vi "Washing_Machine.vi"() -> ()   [LabVIEW 2023]
doc: "This is the main vi that simulates the washing machine."
uses:
  Controls/Wash_Type.ctl
  Controls/Sequence_Display.ctl
  Controls/Washing_Data.ctl
  Controls/Queue_Operation_Select.ctl
  Controls/State_and_Data.ctl
  Controls/Timer_Operation_Select.ctl
  Controls/INI_Operation_Select.ctl
panel:
  out "Sequence":T1
  out "Elapsed_Time":dbl caption="Elapsed Time"
  out "Machine_Underweight":bool
  out "Machine_Overweight":bool
  out "Machine_Load":dbl(slide) caption="Machine Load" scale=0.0..15.0
  in  "Unload":bool
  in  "Stop_Wash":bool caption="Stop Wash"
  in  "Start_Wash":bool caption="Start Wash"
  in  "Wash_Type":T2 caption="Wash Type" scale=0.0..2.0
  in  "Add_Clothes":bool
  in  "Clothes [Kg]":dbl min=0.0 max=15.0
  out "Error_Out":errorcluster
  in  "Error_In":errorcluster
  # "Load Status"
  # "Sec"
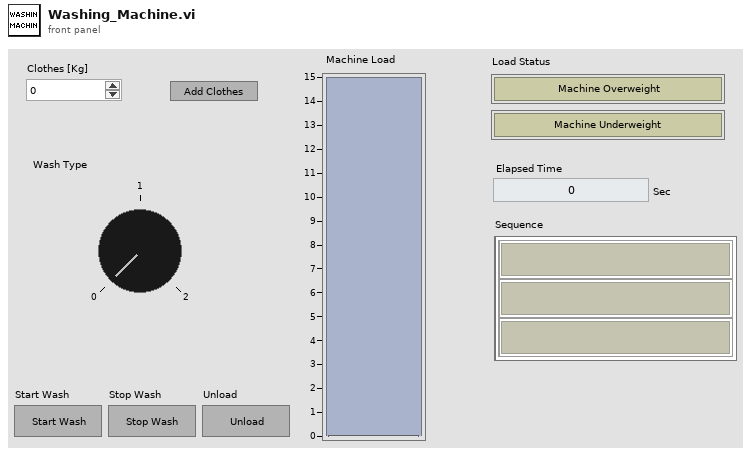
[diagram p1: front panel]
types:
  T1 = typedef "Sequence_Display.ctl" = cluster{"Sequence_LED":bool[], "Sequence_Label":string[]}
  T2 = typedef "Wash_Type.ctl" = i32
  T3 = typedef "Queue_Operation_Select.ctl" = enum16{"Obtain_Queue", "Enqueue", "Enqueue_First", "Enqueue_N", "Lossy_Enqueue", "Preview", "Queue_Status", "Dequeue", "Flush", "Release_Queue"}
  T4 = typedef "State_and_Data.ctl" = cluster{"State":string, "Data":variant}
  T5 = typedef "Washing_Data.ctl" = cluster{"Machine_Load":dbl, "Machine_Overweight":bool, "Machine_Underweight":bool, "Sequence":bool[], "Washing_Complete?":bool, "Disabled":enum8{"Enabled", "Disabled", "Disabled and Grayed Out"}, "Wash_Type":string, "Washing_Process":string[], "Process_Time":dbl[], "CSV_File_Path":path, "Current_Washing_Stage":i32, "Start?":bool, "Total_Washing_Stage":i32, "Washing_Process_F":bool[], "Machine_Load_Added":bool, "Wash_Completed_Time":dbl, "Sequence 2":T1}
  T6 = enum8{"Enabled", "Disabled", "Disabled and Grayed Out"}
  T7 = typedef "INI_Operation_Select.ctl" = enum16{"Initialize", "Read", "Read_Key", "Write"}
  T8 = typedef "Timer_Operation_Select.ctl" = enum16{"Start_Timer", "Time_Out?", "Pause_Timer", "Stop_Timer"}
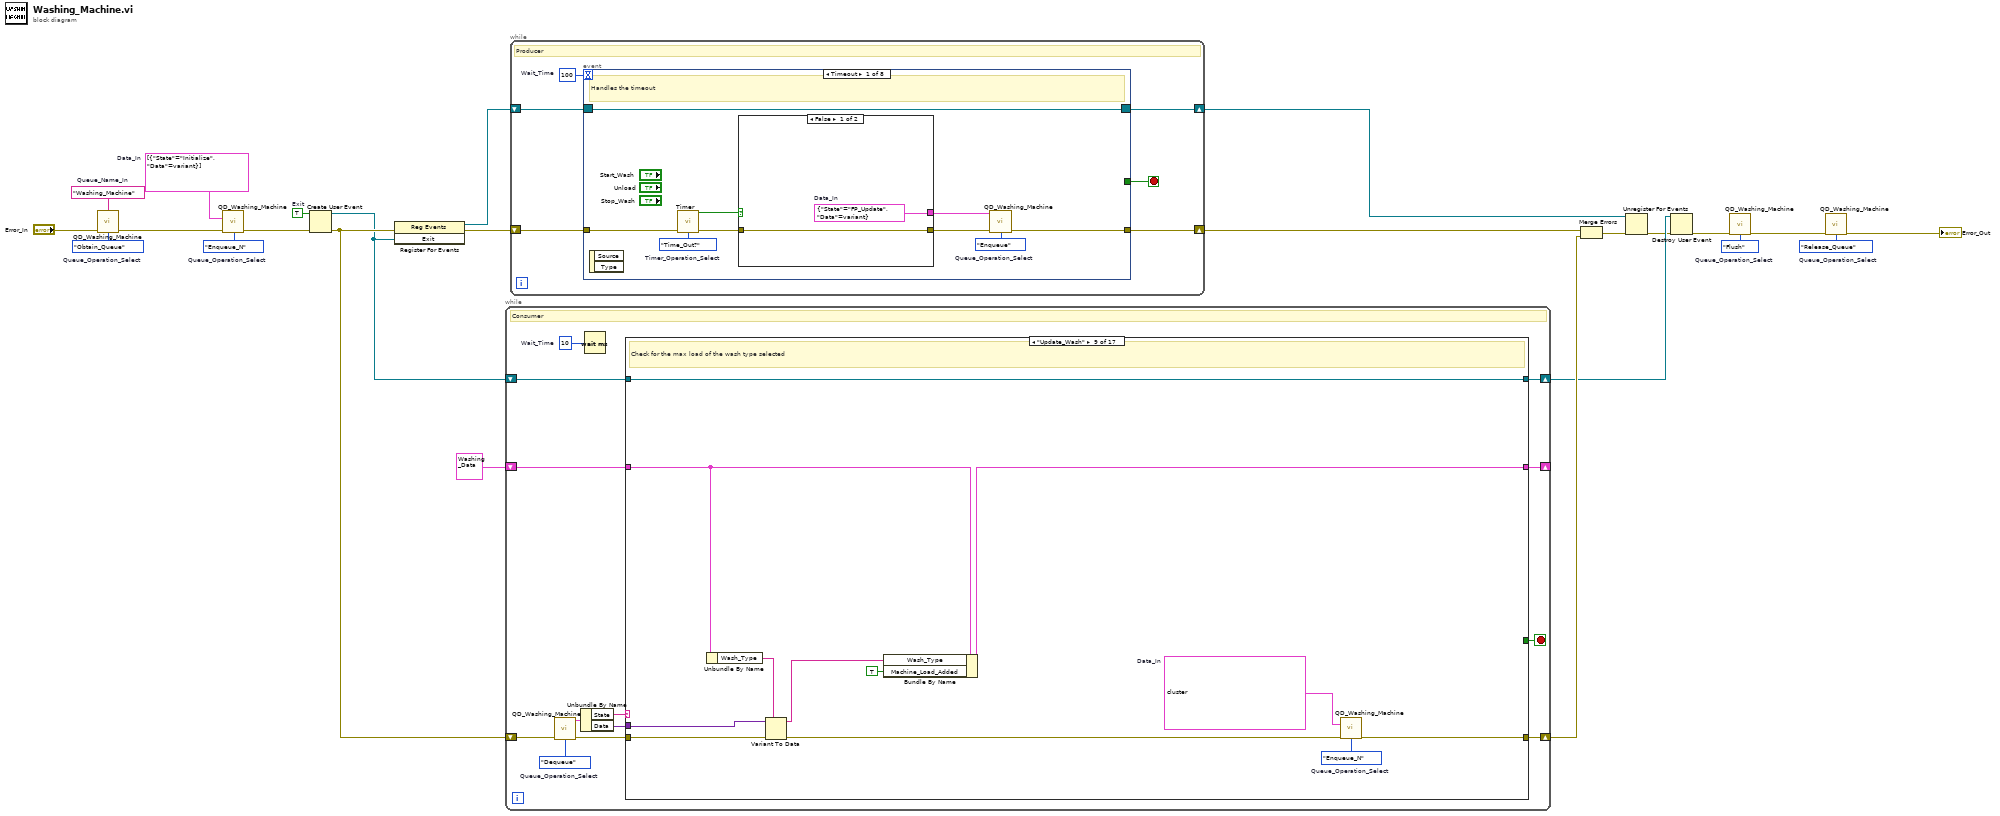
[diagram p0: block diagram]
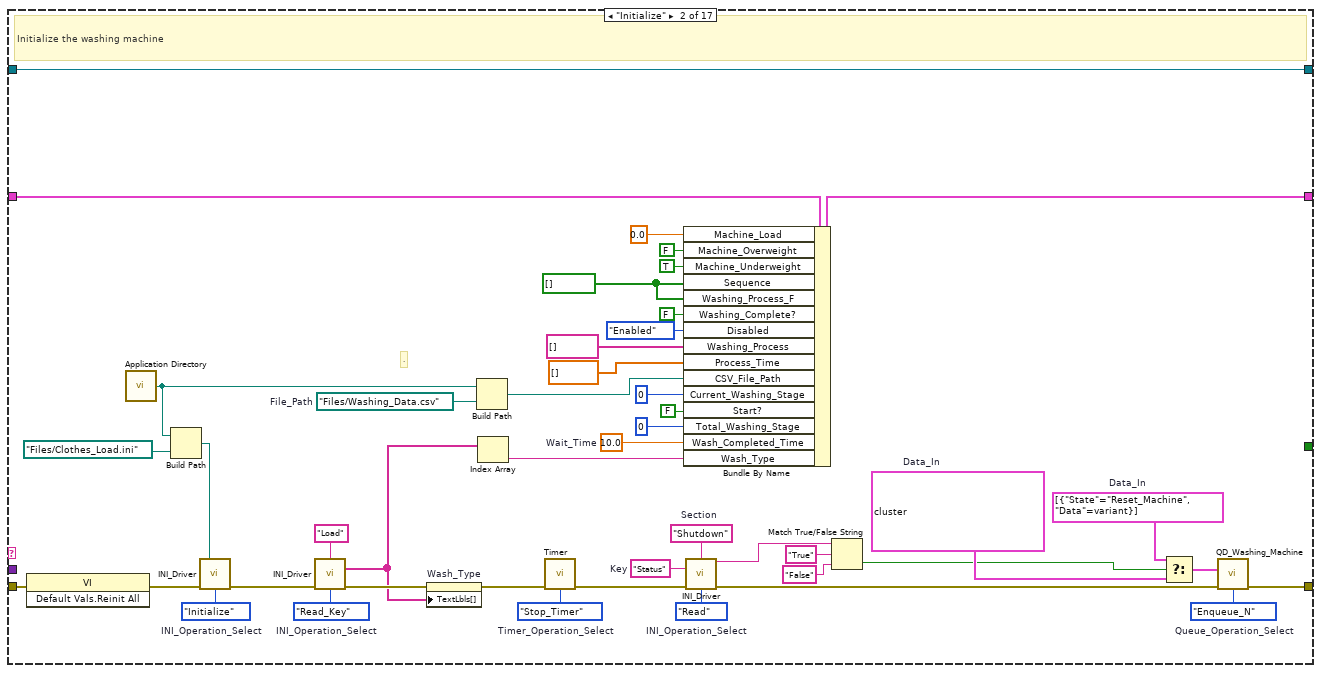
[diagram p3: hidden frame]
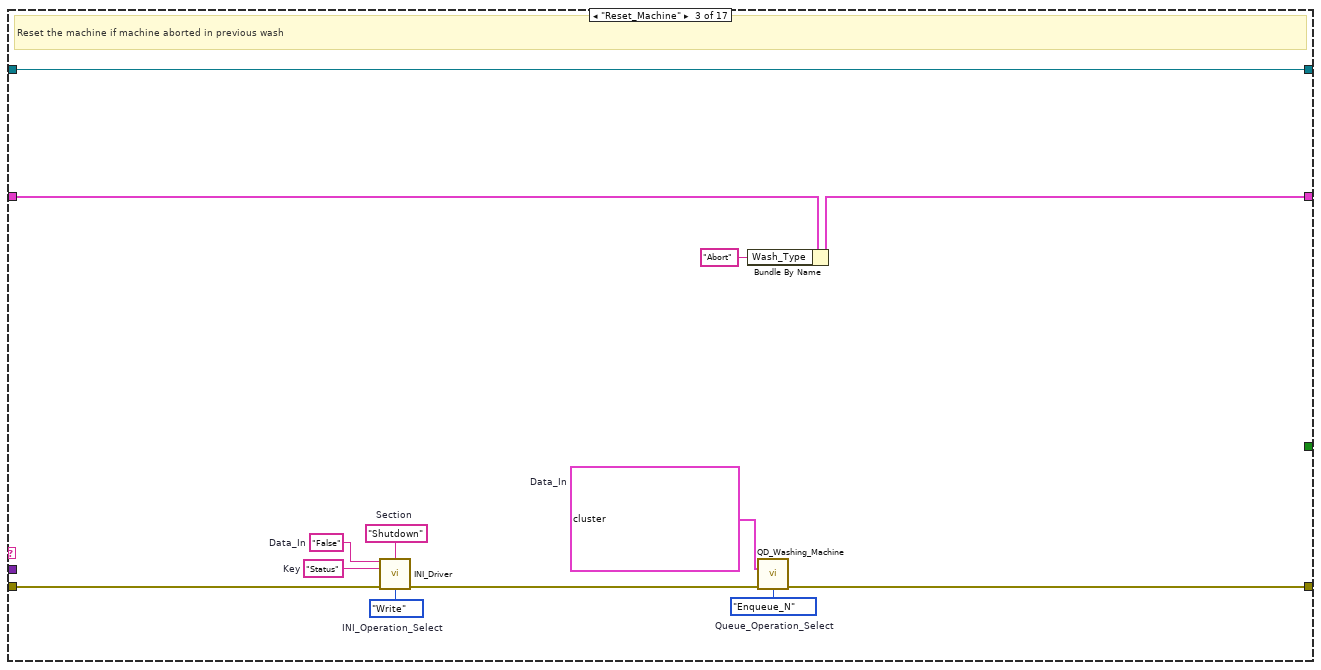
[diagram p4: hidden frame]
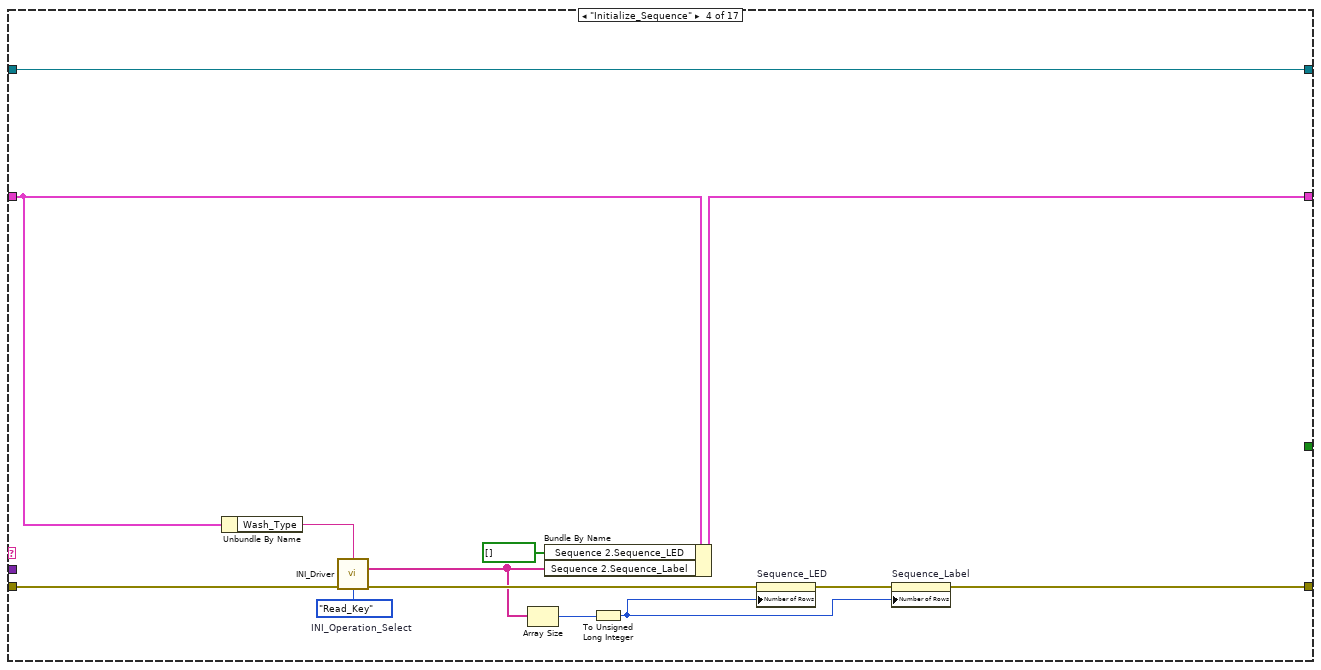
[diagram p5: hidden frame]
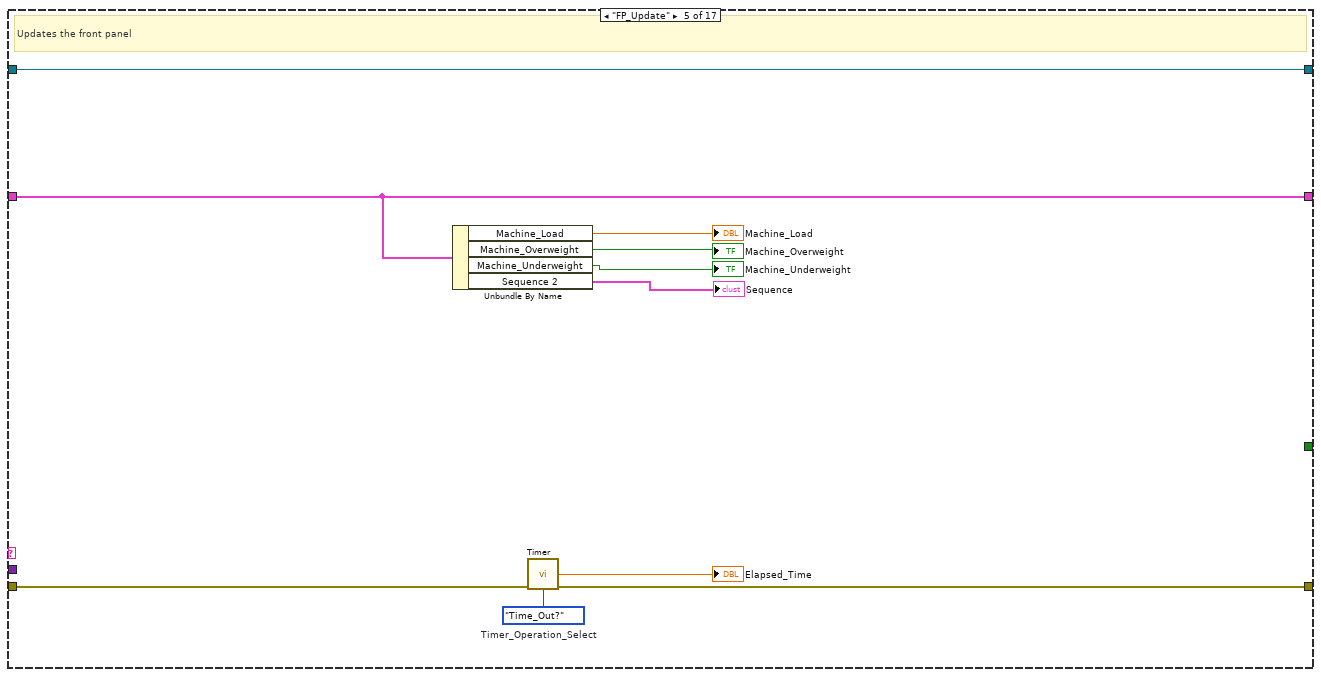
[diagram p6: hidden frame]
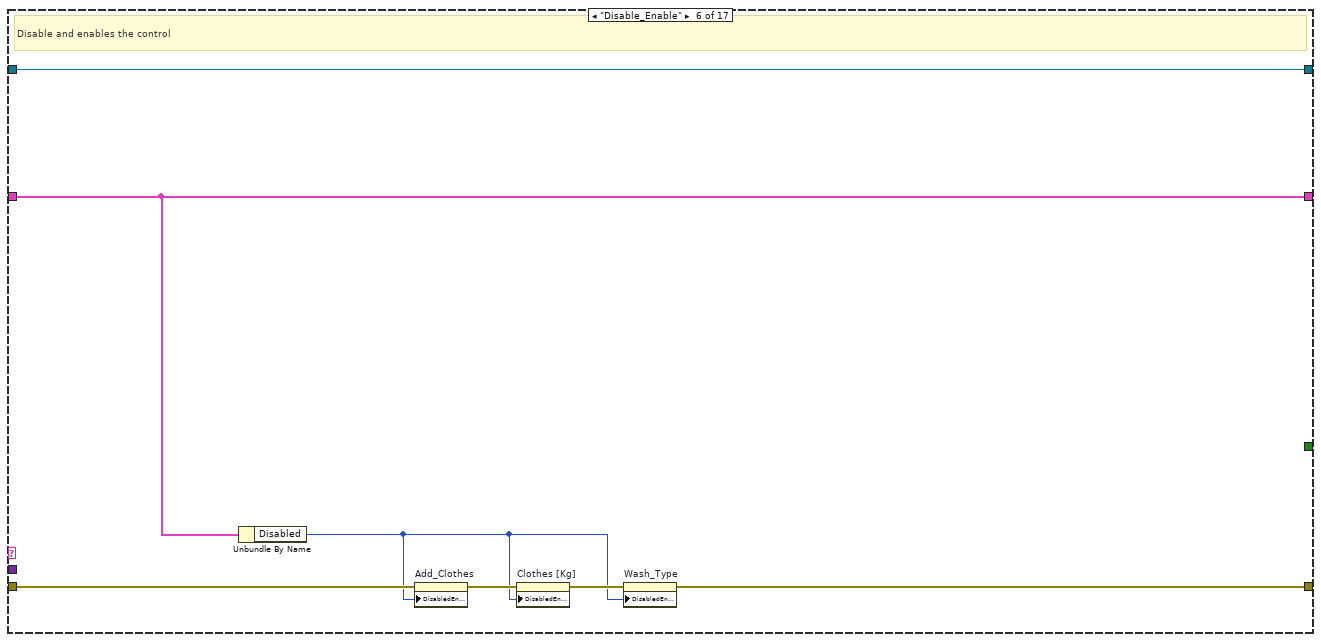
[diagram p7: hidden frame]
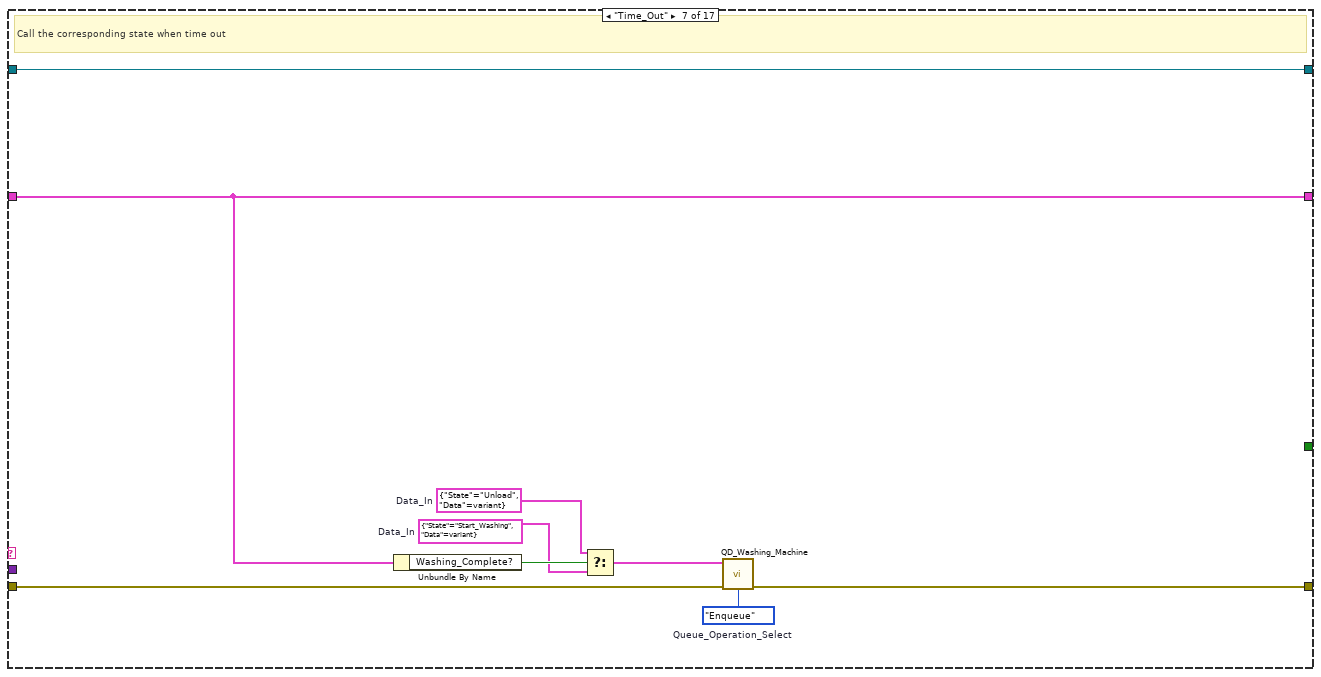
[diagram p8: hidden frame]
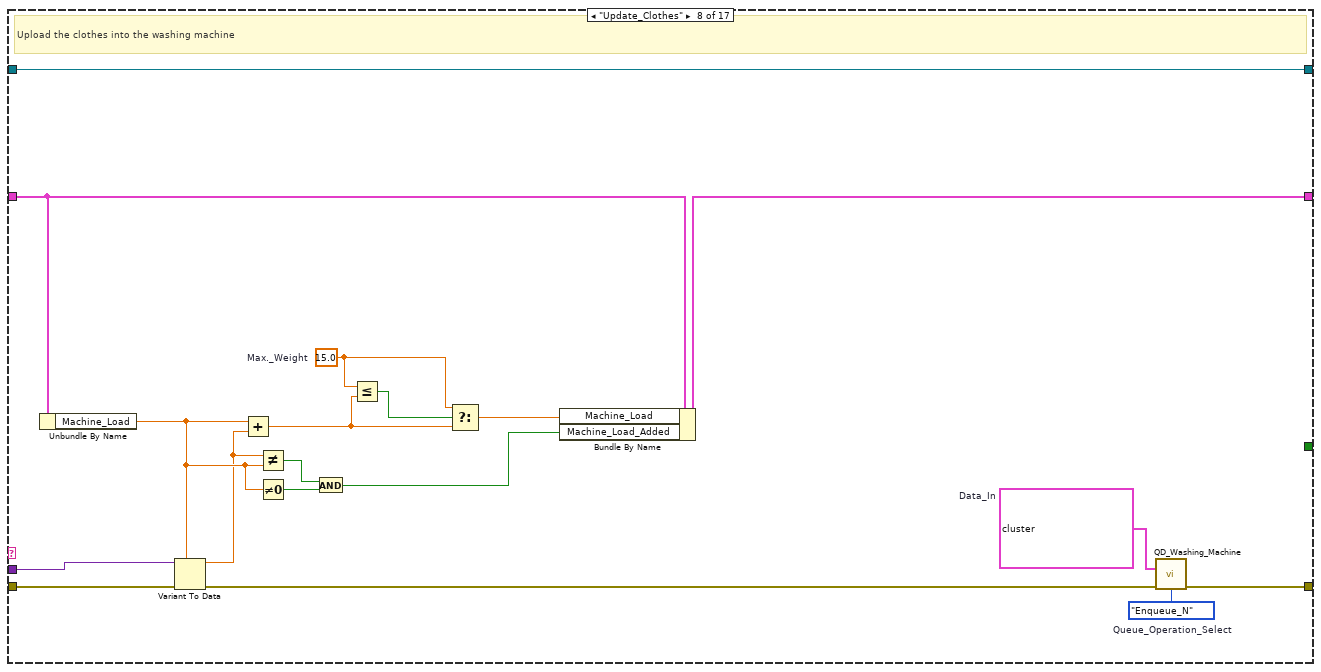
[diagram p9: hidden frame]
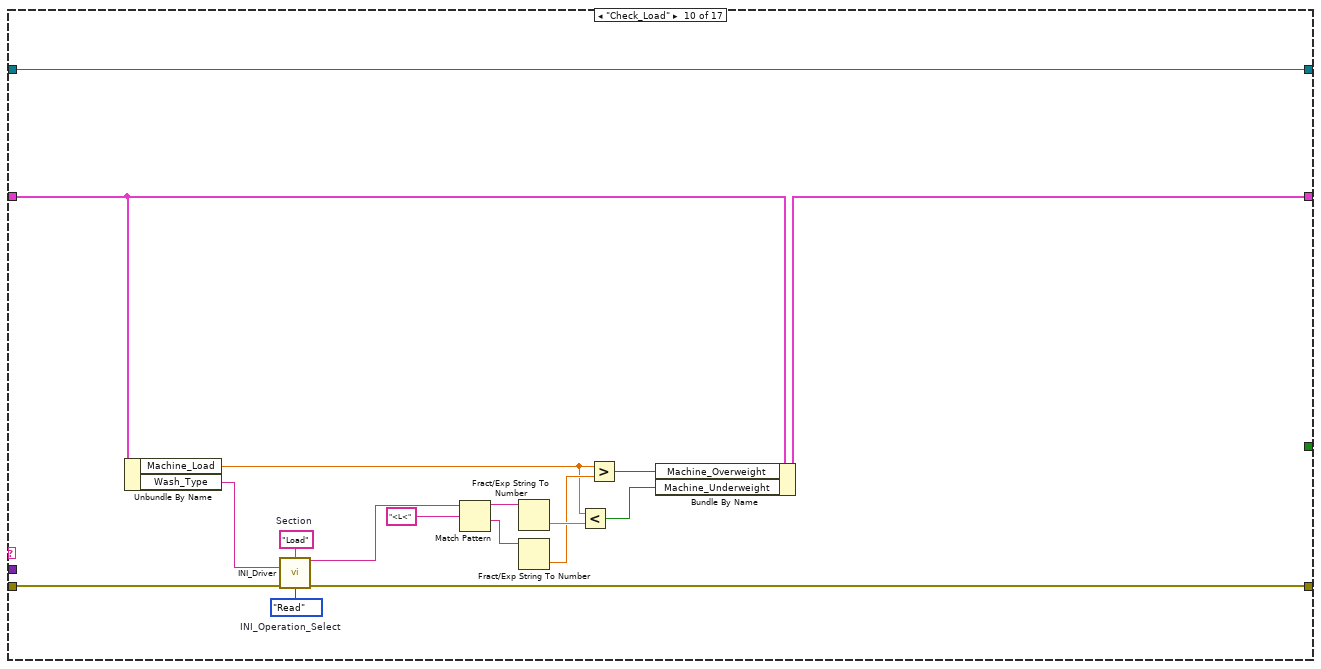
[diagram p10: hidden frame]
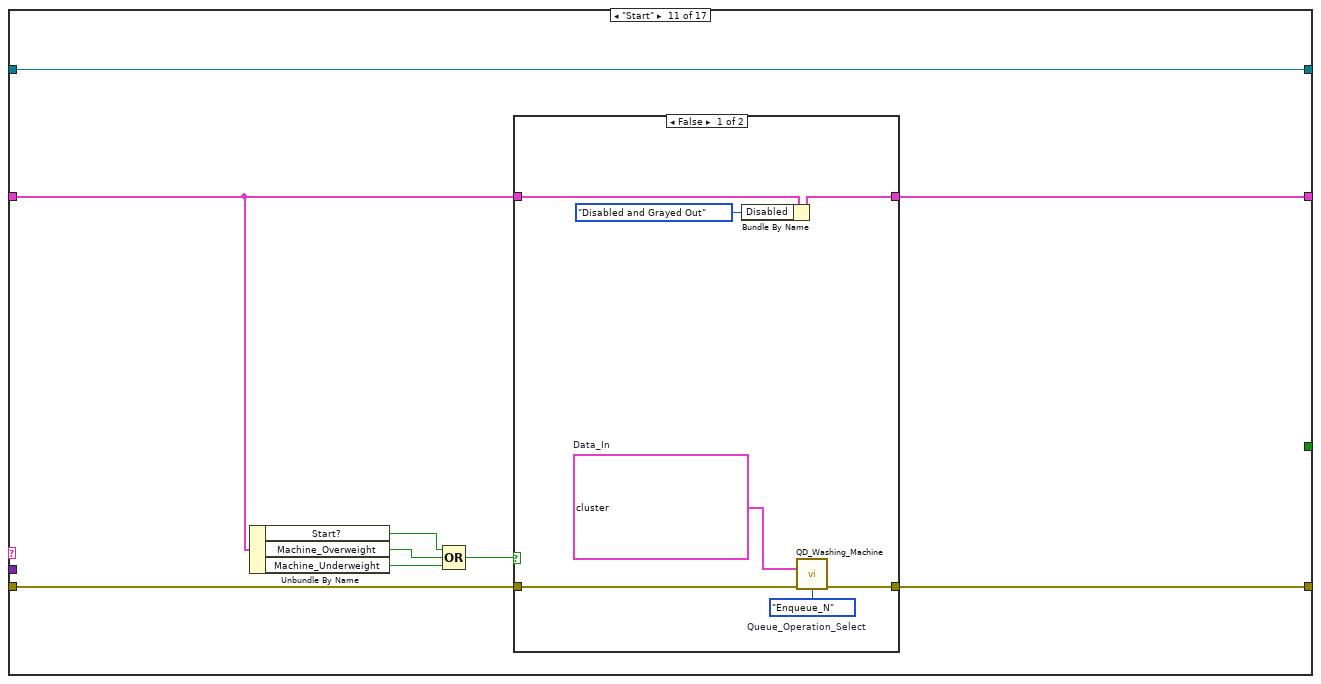
[diagram p11: hidden frame]
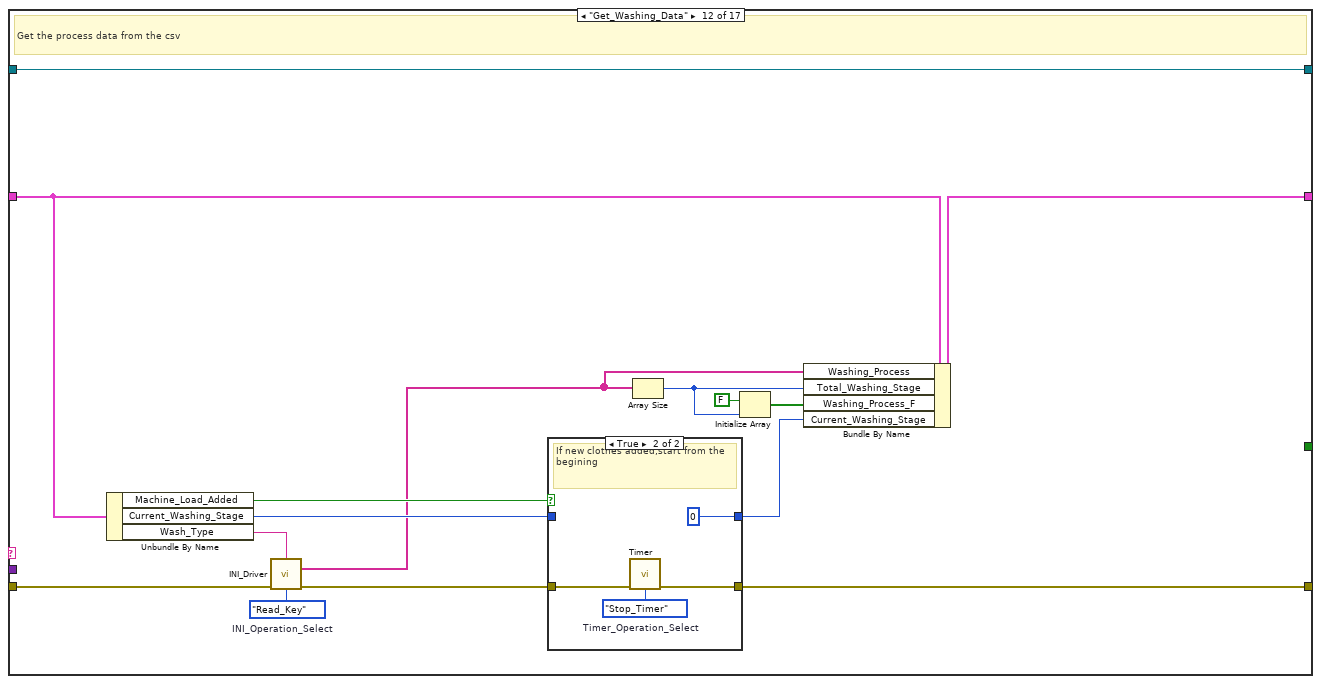
[diagram p13: hidden frame]
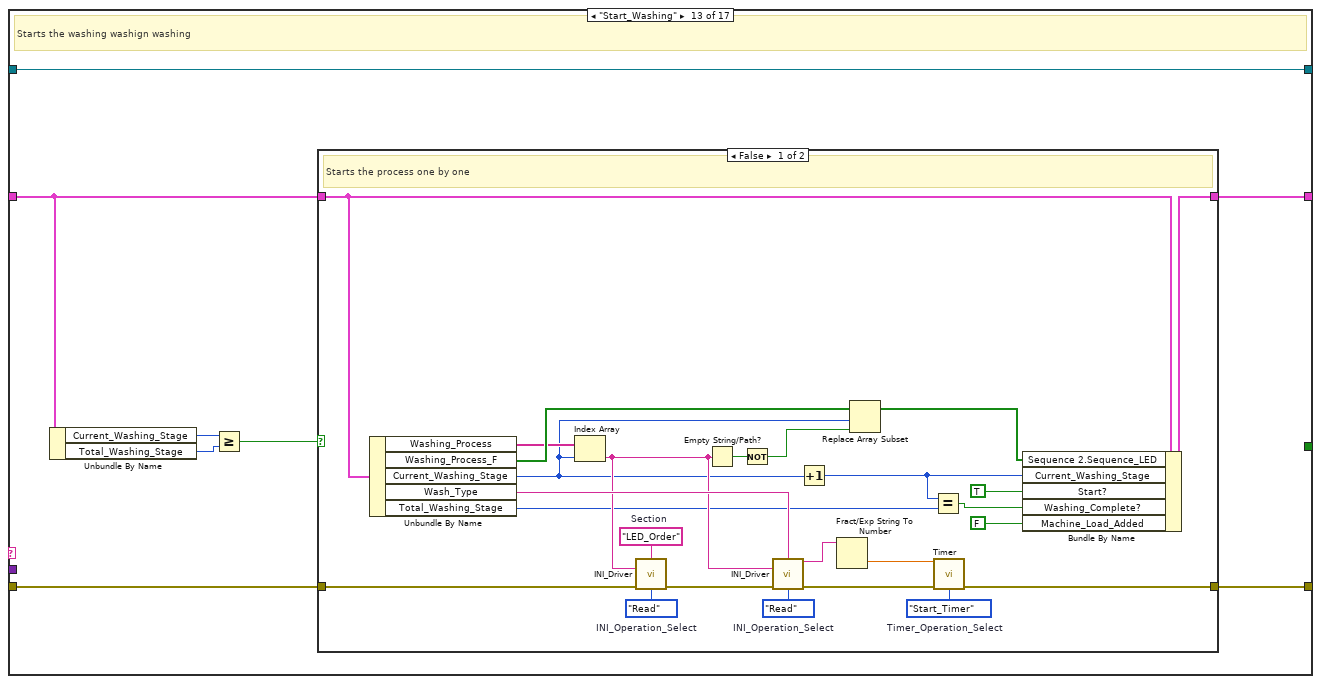
[diagram p15: hidden frame]
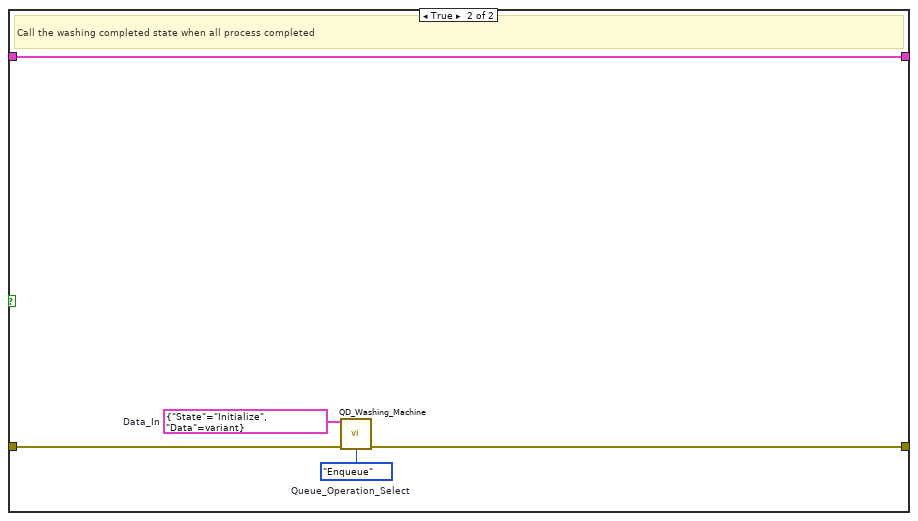
[diagram p16: hidden frame]
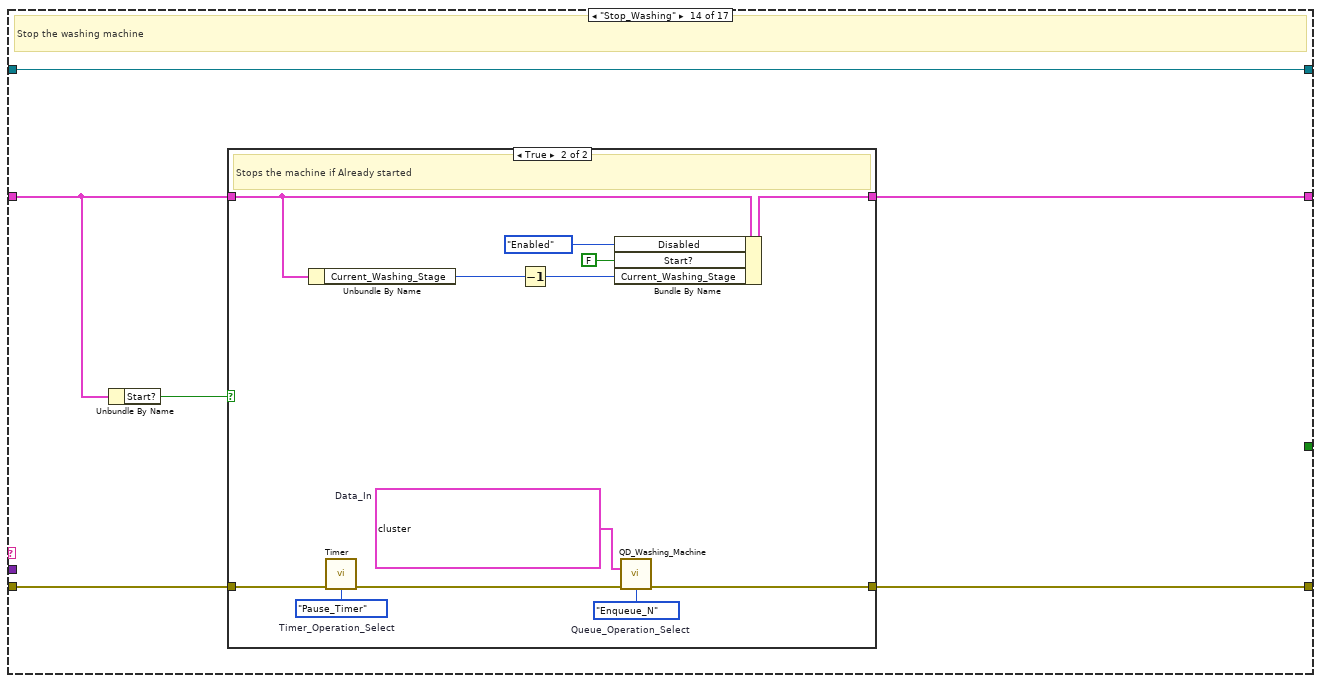
[diagram p17: hidden frame]
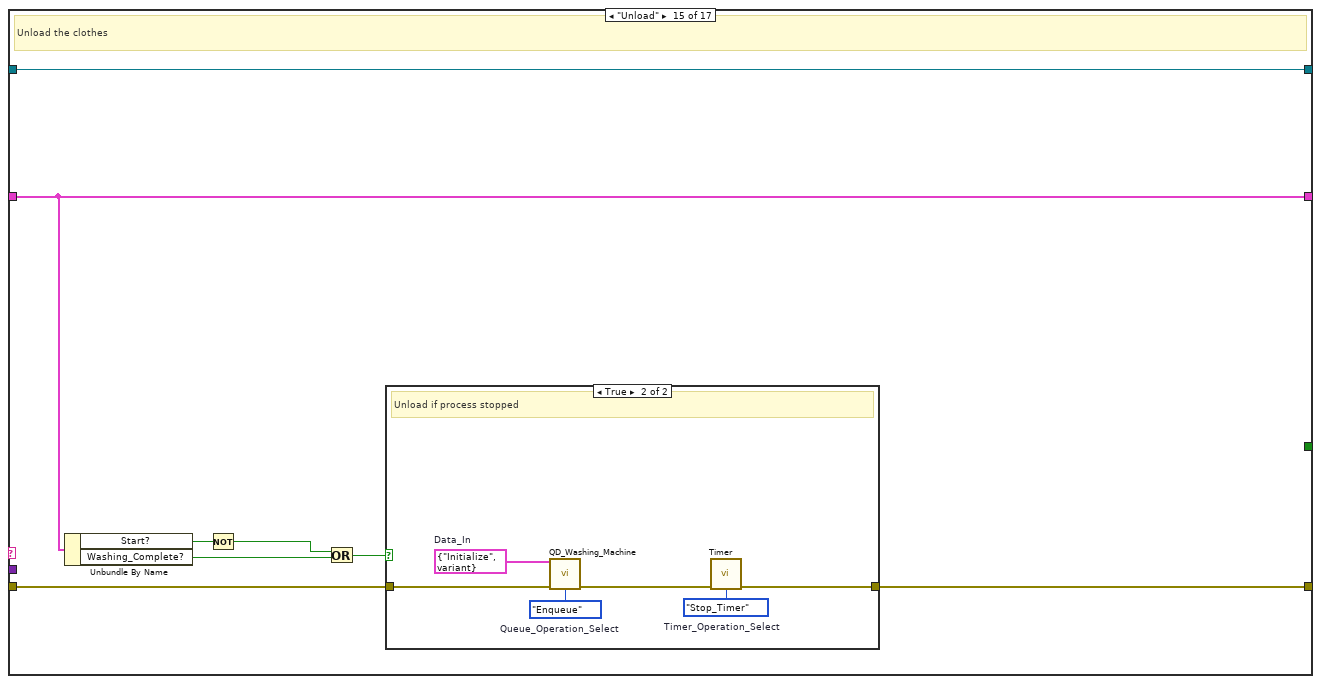
[diagram p19: hidden frame]
diagram:
  w5 = Queue_Operation_Select."Release_Queue"  # Queue_Operation_Select
  w6 = Queue_Operation_Select."Flush"  # Queue_Operation_Select
  w13 = TRUE  # Exit
  w17 = T4[] [{"State"="Initialize", "Data"=variant}]  # Data_In
  w18 = Queue_Operation_Select."Enqueue_N"  # Queue_Operation_Select
  w19 = "Washing_Machine"  # Queue_Name_In
  w20 = Queue_Operation_Select."Obtain_Queue"  # Queue_Operation_Select
  n1 = call "QD_Washing_Machine.vi"("Queue_Name_In"=w19, "Error_In"="Error_In", "Queue_Operation_Select"=w20) -> ("Error_Out"=w22:errorcluster)  [unwired: 10 in, 2 out]
  n2 = call "QD_Washing_Machine.vi"("Data_In"=w17, "Error_In"=w22, "Queue_Operation_Select"=w18) -> ("Error_Out"=w15:errorcluster)  [unwired: 10 in, 2 out]
  n3 = Create User Event(user event datatype=w13, error in=w15) -> (user event=w4:refnum<user-event>, error out=w14:errorcluster)
  n4 = register-events(error in=w14, w4) -> (reference out=w11:refnum<event-registration>, error out=w12:errorcluster)  [unwired: 1 in]
  n5 = while {
    shift-right: [w36] -> w16
    shift-left: w14 -> [w37]
    shift-right: [w30] -> _
    shift-left: T5 {"Machine_Load"=0.0, "Machine_Overweight"=FALSE, "Machine_Underweight"=FALSE, "Sequence"=[], "Washing_Complete?"=FALSE, "Disabled"=enum."Enabled", "Wash_Type"="", "Washing_Process"=[], "Process_Time"=[], "CSV_File_Path"=path "", "Current_Washing_Stage"=0, "Start?"=FALSE, "Total_Washing_Stage"=0, "Washing_Process_F"=[], "Machine_Load_Added"=FALSE, "Wash_Completed_Time"=0.0, "Sequence 2"={"Sequence_LED"=[], "Sequence_Label"=[]}} -> [w29]
    shift-right: [w25] -> w3
    shift-left: w4 -> [w26]
    stop <- w28 stop-if-true
    w27 = u32 10  # Wait_Time
    w34 = Queue_Operation_Select."Dequeue"  # Queue_Operation_Select
    # "Consumer"
    n6 = call "QD_Washing_Machine.vi"("Error_In"=w37, "Queue_Operation_Select"=w34) -> ("Data_Out"=w33:T4, "Error_Out"=w35:errorcluster)  [unwired: 11 in, 1 out]
    n7 = Unbundle By Name(w33) -> ("State"=w32:string, "Data"=w31:variant)
    n8 = Wait (ms)(milliseconds to wait=w27) -> ()  [unwired: 1 out]
    n9 = case shown="\"Update_Wash\"" w32 {
      tunnel: w35 -> [w40 w49 w90 w108 w121 w128 w137 w155 w167 w175 w193 w207 w231 w267 w289 w299 w329]
      tunnel: [w40 w71 w95 w110 w116 w126 w135 w150 w165 w169 w189 w212 w230 w265 w288 w305 w331] -> w36
      tunnel: w31 -> [_ _ _ _ _ _ _ w152 w166 _ _ _ _ _ _ w300 _]
      tunnel: [w39 w84 w97 w101 w120 w124 w136 w154 w159 w170 w187 w216 w229 w266 w287 w319 w330] -> w30
      tunnel: w29 -> [w39 w85 w98 w102 w120 w124 w136 w151 w163 w174 w188 w217 w228 w264 w287 w319 w330]
      tunnel: [_ _ _ _ _ _ _ _ _ _ _ _ _ _ _ _ w332] -> w28
      tunnel: w26 -> [w38 w51 w88 w111 w113 w122 w129 w148 w164 w184 w192 w210 w225 w262 w285 w297 w333]
      tunnel: [w38 w51 w88 w111 w113 w122 w129 w148 w164 w184 w192 w210 w225 w262 w285 w297 w322] -> w25
      frame Default {
      }
      frame "Initialize" {
        w46 = INI_Operation_Select."Read_Key"  # INI_Operation_Select
        w52 = 10.0  # Wait_Time
        w56 = T4[] [{"State"="Reset_Machine", "Data"=variant}]  # Data_In
        w50 = "Status"  # Key
        w60 = "Shutdown"  # Section
        w61 = INI_Operation_Select."Read"  # INI_Operation_Select
        w66 = Timer_Operation_Select."Stop_Timer"  # Timer_Operation_Select
        w67 = INI_Operation_Select."Initialize"  # INI_Operation_Select
        w69 = T4[] [{"State"="Initialize_Sequence", "Data"=variant}, {"State"="Disable_Enable", "Data"=variant}]  # Data_In
        w70 = Queue_Operation_Select."Enqueue_N"  # Queue_Operation_Select
        w75 = path "Files/Washing_Data.csv"  # File_Path
        w68 = bool[] [] ("Sequence")
        # "."
        # "Initialize the washing machine"
        n10 = invoke on="Invoke Node" class="VI" method="Default Vals.Reinit All"(error in=w49) -> (error out=w53:errorcluster)  [unwired: 2 in, 2 out]
        n11 = call <vilib>:"Application Directory.vi"() -> ("Application Directory"=w63:path)
        n12 = Build Path(base path=w63, name or relative path=path "Files/Clothes_Load.ini" ("Config_File_Path")) -> (appended path=w64:path)
        n13 = call "INI_Driver.vi"("Config_File_Path"=w64, "Error_Out"=w53, "INI_Operation_Select"=w67) -> ("Error_Out"=w43:errorcluster)  [unwired: 10 in, 2 out]
        n14 = call "INI_Driver.vi"("Section"="Load", "Error_Out"=w43, "INI_Operation_Select"=w46) -> ("Key_Names"=w44:string[], "Error_Out"=w47:errorcluster)  [unwired: 10 in, 1 out]
        n15 = property on="Wash_Type" class="Knob (strict)"(error in=w47, "TextLbls[]"=w44) -> (error out=w42:errorcluster)  [unwired: 1 in, 1 out]
        n16 = Build Path(base path=w63, name or relative path=w75) -> (appended path=w76:path)
        n17 = Index Array(array=w44) -> (element=w41:string)  [unwired: 1 in]
        n18 = call "Timer.vi"("Error_In"=w42, "Timer_Operation_Select"=w66) -> ("Error_Out"=w65:errorcluster)  [unwired: 10 in, 3 out]
        n19 = Bundle By Name(cluster=w85, "Machine_Load"=0.0, "Machine_Overweight"=FALSE, "Machine_Underweight"=TRUE, "Sequence"=w68, "Washing_Process_F"=w68, "Washing_Complete?"=FALSE, "Disabled"=T6."Enabled", "Washing_Process"=string[] [], "Process_Time"=dbl[] [], "CSV_File_Path"=w76, "Current_Washing_Stage"=0, "Start?"=FALSE, "Total_Washing_Stage"=0, "Wash_Completed_Time"=w52, "Wash_Type"=w41) -> (w84:T5)
        n20 = call "INI_Driver.vi"("Section"=w60, "Key"=w50, "Error_Out"=w65, "INI_Operation_Select"=w61) -> ("Data_Out"=w59:string, "Error_Out"=w54:errorcluster)  [unwired: 9 in, 1 out]
        n21 = Match True/False String(2:"False" ("false string"), 3:"True" ("true string"), 4:w59) -> (0:w55:bool)  [unwired: 1 out]
        n22 = Select(t=w56, s=w55, f=w69) -> (s? t:f=w48:T4[])
        n23 = call "QD_Washing_Machine.vi"("Data_In"=w48, "Error_In"=w54, "Queue_Operation_Select"=w70) -> ("Error_Out"=w71:errorcluster)  [unwired: 10 in, 2 out]
      }
      frame "Reset_Machine" {
        w86 = "False"  # Data_In
        w87 = "Status"  # Key
        w91 = "Shutdown"  # Section
        w92 = INI_Operation_Select."Write"  # INI_Operation_Select
        w93 = T4[] [{"State"="Initialize_Sequence", "Data"=variant}, {"State"="Get_Washing_Data", "Data"=variant}, {"State"="Start_Washing", "Data"=variant}]  # Data_In
        w94 = Queue_Operation_Select."Enqueue_N"  # Queue_Operation_Select
        # "Reset the machine if machine aborted in previous wash"
        n24 = call "INI_Driver.vi"("Data_In"=w86, "Section"=w91, "Key"=w87, "Error_Out"=w90, "INI_Operation_Select"=w92) -> ("Error_Out"=w89:errorcluster)  [unwired: 8 in, 2 out]
        n25 = Bundle By Name(cluster=w98, "Wash_Type"="Abort") -> (w97:T5)
        n26 = call "QD_Washing_Machine.vi"("Data_In"=w93, "Error_In"=w89, "Queue_Operation_Select"=w94) -> ("Error_Out"=w95:errorcluster)  [unwired: 10 in, 2 out]
      }
      frame "Initialize_Sequence" {
        w106 = INI_Operation_Select."Read_Key"  # INI_Operation_Select
        n27 = Unbundle By Name(w102) -> ("Wash_Type"=w105:string)
        n28 = call "INI_Driver.vi"("Section"=w105, "Error_Out"=w108, "INI_Operation_Select"=w106) -> ("Key_Names"=w100:string[], "Error_Out"=w107:errorcluster)  [unwired: 10 in, 1 out]
        n29 = Array Size(array=w100) -> (size(s)=w104:i32)
        n30 = Bundle By Name(cluster=w102, "Sequence 2.Sequence_LED"=bool[] [], "Sequence 2.Sequence_Label"=w100) -> (w101:T5)
        n31 = To Unsigned Long Integer(number=w104) -> (unsigned 32bit integer=w103:u32)
        n32 = property on="Sequence_LED" class="Arr (strict)"(error in=w107, "Number of Rows"=w103) -> (error out=w109:errorcluster)  [unwired: 1 in, 1 out]
        n33 = property on="Sequence_Label" class="Arr (strict)"(error in=w109, "Number of Rows"=w103) -> (error out=w110:errorcluster)  [unwired: 1 in, 1 out]
      }
      frame "FP_Update" {
        w115 = Timer_Operation_Select."Time_Out?"  # Timer_Operation_Select
        # "Updates the front panel"
        n34 = Unbundle By Name(w120) -> ("Machine_Load"=→"Machine_Load":dbl, "Machine_Overweight"=→"Machine_Overweight":bool, "Machine_Underweight"=→"Machine_Underweight":bool, "Sequence 2"=→"Sequence":T1)
        n35 = call "Timer.vi"("Error_In"=w121, "Timer_Operation_Select"=w115) -> ("Time"=→"Elapsed_Time":dbl, "Error_Out"=w116:errorcluster)  [unwired: 10 in, 2 out]
      }
      frame "Disable_Enable" {
        # "Disable and enables the control"
        n36 = Unbundle By Name(w124) -> ("Disabled"=w123:T6)
        n37 = property on="Add_Clothes" class="Bool"(error in=w128, "DisabledEnum"=w123) -> (error out=w125:errorcluster)  [unwired: 1 in, 1 out]
        n38 = property on="Clothes [Kg]" class="DigNum (strict)"(error in=w125, "DisabledEnum"=w123) -> (error out=w127:errorcluster)  [unwired: 1 in, 1 out]
        n39 = property on="Wash_Type" class="Knob (strict)"(error in=w127, "DisabledEnum"=w123) -> (error out=w126:errorcluster)  [unwired: 1 in, 1 out]
      }
      frame "Time_Out" {
        w131 = T4 {"State"="Start_Washing", "Data"=variant}  # Data_In
        w132 = T4 {"State"="Unload", "Data"=variant}  # Data_In
        w134 = Queue_Operation_Select."Enqueue"  # Queue_Operation_Select
        # "Call the corresponding state when time out"
        n40 = Unbundle By Name(w136) -> ("Washing_Complete?"=w133:bool)
        n41 = Select(t=w132, s=w133, f=w131) -> (s? t:f=w130:T4)
        n42 = call "QD_Washing_Machine.vi"("Data_In"=w130, "Error_In"=w137, "Queue_Operation_Select"=w134) -> ("Error_Out"=w135:errorcluster)  [unwired: 10 in, 2 out]
      }
      frame "Update_Clothes" {
        w138 = 15.0  # Max._Weight
        w142 = T4[] [{"State"="Check_Load", "Data"=variant}, {"State"="FP_Update", "Data"=variant}]  # Data_In
        w149 = Queue_Operation_Select."Enqueue_N"  # Queue_Operation_Select
        # "Upload the clothes into the washing machine"
        n43 = Unbundle By Name(w151) -> ("Machine_Load"=w144:dbl)
        n44 = Variant To Data(error in=w155, type=w144, Variant=w152) -> (data=w143:dbl, error out=w153:errorcluster)
        n45 = Add(x=w144, y=w143) -> (x+y=w139:dbl)
        n46 = Not Equal?(x=w143, y=w144) -> (x != y?=w146:bool)
        n47 = Not Equal To 0?(x=w144) -> (x != 0?=w147:bool)
        n48 = And(x=w146, y=w147) -> (x .and. y?=w145:bool)
        n49 = Less Or Equal?(x=w138, y=w139) -> (x <= y?=w140:bool)
        n50 = Select(t=w138, s=w140, f=w139) -> (s? t:f=w141:dbl)
        n51 = Bundle By Name(cluster=w151, "Machine_Load"=w141, "Machine_Load_Added"=w145) -> (w154:T5)
        n52 = call "QD_Washing_Machine.vi"("Data_In"=w142, "Error_In"=w153, "Queue_Operation_Select"=w149) -> ("Error_Out"=w150:errorcluster)  [unwired: 10 in, 2 out]
      }
      frame "Update_Wash" {
        w157 = T4[] [{"State"="Initialize_Sequence", "Data"=variant}, {"State"="Check_Load", "Data"=variant}, {"State"="FP_Update", "Data"=variant}]  # Data_In
        w161 = Queue_Operation_Select."Enqueue_N"  # Queue_Operation_Select
        # "Check for the max load of the wash type selected"
        n53 = Unbundle By Name(w163) -> ("Wash_Type"=w162:string)
        n54 = Variant To Data(error in=w167, type=w162, Variant=w166) -> (data=w160:string, error out=w158:errorcluster)
        n55 = Bundle By Name(cluster=w163, "Wash_Type"=w160, "Machine_Load_Added"=TRUE) -> (w159:T5)
        n56 = call "QD_Washing_Machine.vi"("Data_In"=w157, "Error_In"=w158, "Queue_Operation_Select"=w161) -> ("Error_Out"=w165:errorcluster)  [unwired: 10 in, 2 out]
      }
      frame "Check_Load" {
        w176 = "Load"  # Section
        w177 = INI_Operation_Select."Read"  # INI_Operation_Select
        n57 = Unbundle By Name(w174) -> ("Machine_Load"=w173:dbl, "Wash_Type"=w168:string)
        n58 = call "INI_Driver.vi"("Section"=w176, "Key"=w168, "Error_Out"=w175, "INI_Operation_Select"=w177) -> ("Data_Out"=w183:string, "Error_Out"=w169:errorcluster)  [unwired: 9 in, 1 out]
        n59 = Match Pattern(string=w183, regular expression="<L<") -> (before substring=w181:string, after substring=w180:string)  [unwired: 1 in, 2 out]
        n60 = Fract/Exp String To Number(string=w181) -> (number=w179:dbl)  [unwired: 3 in, 1 out]
        n61 = Fract/Exp String To Number(string=w180) -> (number=w178:dbl)  [unwired: 3 in, 1 out]
        n62 = Less?(x=w173, y=w179) -> (x < y?=w171:bool)
        n63 = Greater?(x=w173, y=w178) -> (0:w172:bool)
        n64 = Bundle By Name(cluster=w174, "Machine_Overweight"=w172, "Machine_Underweight"=w171) -> (w170:T5)
      }
      frame "Start" {
        n65 = Unbundle By Name(w188) -> ("Start?"=w186:bool, "Machine_Overweight"=w190:bool, "Machine_Underweight"=w191:bool)
        n66 = Compound Arithmetic op=OR(w186, w190, w191) -> (w185:bool)
        n67 = case shown="False" w185 {
          tunnel: w193 -> [w200 w202]
          tunnel: [w199 w202] -> w189
          tunnel: w188 -> [w196 w201]
          tunnel: [w195 w201] -> w187
          frame False {
            w197 = T4[] [{"State"="Disable_Enable", "Data"=variant}, {"State"="Get_Washing_Data", "Data"=variant}, {"State"="Start_Washing", "Data"=variant}]  # Data_In
            w198 = Queue_Operation_Select."Enqueue_N"  # Queue_Operation_Select
            n68 = Bundle By Name(cluster=w196, "Disabled"=T6."Disabled and Grayed Out") -> (w195:T5)
            n69 = call "QD_Washing_Machine.vi"("Data_In"=w197, "Error_In"=w200, "Queue_Operation_Select"=w198) -> ("Error_Out"=w199:errorcluster)  [unwired: 10 in, 2 out]
          }
          frame True {
          }
        }
      }
      frame "Get_Washing_Data" {
        w205 = INI_Operation_Select."Read_Key"  # INI_Operation_Select
        # "Get the process data from the csv"
        n70 = Unbundle By Name(w217) -> ("Machine_Load_Added"=w211:bool, "Current_Washing_Stage"=w209:i32, "Wash_Type"=w203:string)
        n71 = call "INI_Driver.vi"("Section"=w203, "Error_Out"=w207, "INI_Operation_Select"=w205) -> ("Key_Names"=w204:string[], "Error_Out"=w206:errorcluster)  [unwired: 10 in, 1 out]
        n72 = case shown="True" w211 {
          tunnel: w206 -> [w219 w223]
          tunnel: [w219 w222] -> w212
          tunnel: w209 -> [w218 _]
          tunnel: [w218 0 ("Current_Washing_Stage")] -> w208
          frame False {
          }
          frame True {
            w221 = Timer_Operation_Select."Stop_Timer"  # Timer_Operation_Select
            # "If new clothes added,start from the begining"
            n73 = call "Timer.vi"("Error_In"=w223, "Timer_Operation_Select"=w221) -> ("Error_Out"=w222:errorcluster)  [unwired: 10 in, 3 out]
          }
        }
        n74 = Array Size(array=w204) -> (size(s)=w214:i32)
        n75 = Initialize Array(FALSE ("Sequence"), w214) -> (w215:bool[])
        n76 = Bundle By Name(cluster=w217, "Washing_Process"=w204, "Total_Washing_Stage"=w214, "Washing_Process_F"=w215, "Current_Washing_Stage"=w208) -> (w216:T5)
      }
      frame "Start_Washing" {
        # "Starts the washing washign washing"
        n77 = Unbundle By Name(w228) -> ("Current_Washing_Stage"=w227:i32, "Total_Washing_Stage"=w226:i32)
        n78 = Greater Or Equal?(x=w227, y=w226) -> (x >= y?=w224:bool)
        n79 = case shown="False" w224 {
          tunnel: w231 -> [w256 w260]
          tunnel: w228 -> [w255 w261]
          tunnel: [w254 w259] -> w230
          tunnel: [w252 w261] -> w229
          frame False {
            w238 = "LED_Order"  # Section
            w240 = INI_Operation_Select."Read"  # INI_Operation_Select
            w245 = INI_Operation_Select."Read"  # INI_Operation_Select
            w253 = Timer_Operation_Select."Start_Timer"  # Timer_Operation_Select
            # "Starts the process one by one"
            n80 = Unbundle By Name(w255) -> ("Washing_Process"=w249:string[], "Washing_Process_F"=w251:bool[], "Current_Washing_Stage"=w236:i32, "Wash_Type"=w244:string, "Total_Washing_Stage"=w233:i32)
            n81 = Index Array(array=w249, index=w236) -> (element=w239:string)
            n82 = call "INI_Driver.vi"("Section"=w238, "Key"=w239, "Error_Out"=w256, "INI_Operation_Select"=w240) -> ("Error_Out"=w241:errorcluster)  [unwired: 9 in, 2 out]
            n83 = Empty String/Path?(string/path=w239) -> (empty?=w248:bool)
            n84 = Not(x=w248) -> (.not. x?=w247:bool)
            n85 = call "INI_Driver.vi"("Section"=w244, "Key"=w239, "Error_Out"=w241, "INI_Operation_Select"=w245) -> ("Data_Out"=w243:string, "Error_Out"=w246:errorcluster)  [unwired: 9 in, 1 out]
            n86 = Increment(x=w236) -> (x+1=w234:i32)
            n87 = Fract/Exp String To Number(string=w243) -> (number=w242:dbl)  [unwired: 3 in, 1 out]
            n88 = Replace Array Subset(array=w251, new element=w247, index=w236) -> (w237:bool[])
            n89 = Equal?(x=w234, y=w233) -> (x = y?=w232:bool)
            n90 = call "Timer.vi"("Wait_Time"=w242, "Error_In"=w246, "Timer_Operation_Select"=w253) -> ("Error_Out"=w254:errorcluster)  [unwired: 9 in, 3 out]
            n91 = Bundle By Name(cluster=w255, "Sequence 2.Sequence_LED"=w237, "Current_Washing_Stage"=w234, "Start?"=TRUE, "Washing_Complete?"=w232, "Machine_Load_Added"=FALSE) -> (w252:T5)
          }
          frame True {
            w257 = Queue_Operation_Select."Enqueue"  # Queue_Operation_Select
            w258 = T4 {"State"="Initialize", "Data"=variant}  # Data_In
            # "Call the washing completed state when all process completed"
            n92 = call "QD_Washing_Machine.vi"("Data_In"=w258, "Error_In"=w260, "Queue_Operation_Select"=w257) -> ("Error_Out"=w259:errorcluster)  [unwired: 10 in, 2 out]
          }
        }
      }
      frame "Stop_Washing" {
        # "Stop the washing machine"
        n93 = Unbundle By Name(w264) -> ("Start?"=w263:bool)
        n94 = case shown="True" w263 {
          tunnel: w267 -> [w268 w281]
          tunnel: [w269 w280] -> w266
          tunnel: [w268 w276] -> w265
          tunnel: w264 -> [w269 w272]
          frame False {
          }
          frame True {
            w274 = T4[] [{"State"="Disable_Enable", "Data"=variant}, {"State"="FP_Update", "Data"=variant}]  # Data_In
            w275 = Queue_Operation_Select."Enqueue_N"  # Queue_Operation_Select
            w277 = Timer_Operation_Select."Pause_Timer"  # Timer_Operation_Select
            # "Stops the machine if Already started"
            n95 = Unbundle By Name(w272) -> ("Current_Washing_Stage"=w271:i32)
            n96 = call "Timer.vi"("Error_In"=w281, "Timer_Operation_Select"=w277) -> ("Error_Out"=w278:errorcluster)  [unwired: 10 in, 3 out]
            n97 = Decrement(x=w271) -> (x-1=w270:i32)
            n98 = Bundle By Name(cluster=w272, "Disabled"=T6."Enabled", "Start?"=FALSE, "Current_Washing_Stage"=w270) -> (w280:T5)
            n99 = call "QD_Washing_Machine.vi"("Data_In"=w274, "Error_In"=w278, "Queue_Operation_Select"=w275) -> ("Error_Out"=w276:errorcluster)  [unwired: 10 in, 2 out]
          }
        }
      }
      frame "Unload" {
        # "Unload the clothes"
        n100 = Unbundle By Name(w287) -> ("Start?"=w283:bool, "Washing_Complete?"=w286:bool)
        n101 = Not(x=w283) -> (.not. x?=w282:bool)
        n102 = Or(x=w282, y=w286) -> (x .or. y?=w284:bool)
        n103 = case shown="True" w284 {
          tunnel: w289 -> [w290 w296]
          tunnel: [w290 w292] -> w288
          frame False {
          }
          frame True {
            w291 = Timer_Operation_Select."Stop_Timer"  # Timer_Operation_Select
            w293 = T4 {"State"="Initialize", "Data"=variant}  # Data_In
            w294 = Queue_Operation_Select."Enqueue"  # Queue_Operation_Select
            # "Unload if process stopped"
            n104 = call "QD_Washing_Machine.vi"("Data_In"=w293, "Error_In"=w296, "Queue_Operation_Select"=w294) -> ("Error_Out"=w295:errorcluster)  [unwired: 10 in, 2 out]
            n105 = call "Timer.vi"("Error_In"=w295, "Timer_Operation_Select"=w291) -> ("Error_Out"=w292:errorcluster)  [unwired: 10 in, 3 out]
          }
        }
      }
      frame "Error" {
        w303 = Queue_Operation_Select."Enqueue"  # Queue_Operation_Select
        w313 = "%d%s%s"  # Format_String
        w312 = "Application Error"  # Initial_String
        w309 = "Stop"  # T_Button
        w310 = "Continue"  # F_Button
        # "Handle the Error"
        n106 = Variant To Data(error in=w299, type=w299, Variant=w300) -> (data=w298:errorcluster, error out=w301:errorcluster)
        n107 = Unbundle By Name(w298) -> ("code"=w315:i32, "source"=w316:string)
        n108 = Format Into String(format string=w313, initial string=w312, error in=w301, w315, "\n" ("Line Feed Constant"), w316) -> (resulting string=w314:string, error out=w306:errorcluster)
        n109 = Two Button Dialog(message=w314, 1:w310, 2:w309) -> (T button?=w317:bool)
        n110 = Select(t="Exit" ("State"), s=w317, f="" ("Empty String Constant")) -> (s? t:f=w318:string)
        n111 = Bundle By Name(cluster=T4 {"State"="", "Data"=variant} ("Data_In"), "State"=w318) -> (w304:T4)
        n112 = call "QD_Washing_Machine.vi"("Data_In"=w304, "Error_In"=w306, "Queue_Operation_Select"=w303) -> ("Error_Out"=w305:errorcluster)  [unwired: 10 in, 2 out]
      }
      frame "Exit" {
        w323 = "Shutdown"  # Section
        w321 = "Status"  # Key
        w324 = INI_Operation_Select."Write"  # INI_Operation_Select
        w332 = TRUE  # Exit
        # "Handles the request for Exit"
        n113 = Unbundle By Name(w330) -> ("Start?"=w328:bool)
        n114 = case shown="False" w328 {
          tunnel: w329 -> [w336 w342]
          tunnel: [w336 w342] -> w327
          tunnel: [w335 w338] -> w326
          tunnel: [w334 w337] -> w320
          frame False {
            w334 = "False"  # Data
            w335 = TRUE  # Exit
          }
          frame True {
            w337 = "True"  # Data
            w339 = "No"  # Continue
            w340 = "Yes"  # Stop
            w341 = "Do you want to Exit"  # Message
            n115 = Two Button Dialog(message=w341, 1:w339, 2:w340) -> (T button?=w338:bool)
          }
        }
        n116 = call "INI_Driver.vi"("Data_In"=w320, "Section"=w323, "Key"=w321, "Error_Out"=w327, "INI_Operation_Select"=w324) -> ("Error_Out"=w325:errorcluster)  [unwired: 8 in, 2 out]
        n117 = Generate User Event(user event=w333, event data cluster=w326, error in=w325) -> (user event out=w322:refnum<user-event>, error out=w331:errorcluster)  [unwired: 1 in]
      }
    }
  }
  n118 = while {
    shift-right: [w348] -> w23
    shift-left: w12 -> [w347]
    shift-right: [w343] -> w1
    shift-left: w11 -> [w344]
    stop <- w346 stop-if-true
    w345 = 100  # Wait_Time
    # "Producer"
    n119 = event shown="[0] Timeout" {
      selector: w344 -> [w349 w364 w375 w389 w397 w405 w413 w424]
      dyn-events: [w349 w364 w375 w389 w397 w405 w413 w424] -> w343
      timeout: w345 -> [_ _ _ _ _ _ _ _]
      tunnel: [w356 w372 w374 w395 w398 w411 w420 w423] -> w348
      tunnel: w347 -> [w357 w373 w388 w396 w404 w412 w421 w423]
      tunnel: [_ FALSE FALSE FALSE FALSE FALSE FALSE w422] -> w346
      event Timeout {
        w354 = Timer_Operation_Select."Time_Out?"  # Timer_Operation_Select
        w355 = Queue_Operation_Select."Enqueue"  # Queue_Operation_Select
        # "Handles the timeout"
        n120 = event-data() -> ()  [unwired: 1 in, 2 out]
        n121 = call "Timer.vi"("Error_In"=w357, "Timer_Operation_Select"=w354) -> ("Time_Out?"=w352:bool, "Error_Out"=w350:errorcluster)  [unwired: 10 in, 2 out]
        n122 = case shown="False" w352 {
          tunnel: [w358 w363] -> w353
          tunnel: [w359 w361] -> w351
          tunnel: w350 -> [w359 w362]
          frame False {
            w358 = T4 {"State"="FP_Update", "Data"=variant}  # Data_In
          }
          frame True {
            w360 = Timer_Operation_Select."Stop_Timer"  # Timer_Operation_Select
            w363 = T4 {"State"="Time_Out", "Data"=variant}  # Data_In
            # "Call the Timeout event when timer timeout happens"
            n123 = call "Timer.vi"("Error_In"=w362, "Timer_Operation_Select"=w360) -> ("Error_Out"=w361:errorcluster)  [unwired: 10 in, 3 out]
          }
        }
        n124 = call "QD_Washing_Machine.vi"("Data_In"=w353, "Error_In"=w351, "Queue_Operation_Select"=w355) -> ("Error_Out"=w356:errorcluster)  [unwired: 10 in, 2 out]
      }
      event "Add_Clothes": Value Change {
        w371 = Queue_Operation_Select."Enqueue"  # Queue_Operation_Select
        # "Add the clothes to machine"
        n125 = event-data() -> ()  [unwired: 1 in, 1 out]
        n126 = To Variant(anything="Clothes [Kg]") -> (Variant=w366:variant)
        n127 = Bundle By Name(cluster=T4 {"State"="", "Data"=variant} ("State_and_Data"), "State"="Update_Clothes", "Data"=w366) -> (w368:T4)
        n128 = call "QD_Washing_Machine.vi"("Data_In"=w368, "Error_In"=w373, "Queue_Operation_Select"=w371) -> ("Error_Out"=w372:errorcluster)  [unwired: 10 in, 2 out]
      }
      event Value Change {
        w376 = 0  # Data_Type
        w387 = Queue_Operation_Select."Enqueue"  # Queue_Operation_Select
        # "Request to start the washing process"
        n129 = event-data() -> ()  [unwired: 1 in, 1 out]
        n130 = property on="Wash_Type" class="Knob (strict)"(error in=w388) -> (error out=w381:errorcluster, "TextLbls[]"=w380:string[], "Value"=w378:T2)  [unwired: 1 in, 1 out]
        n131 = Coerce To Type(0:w378, 1:w376) -> (2:w377:i32)
        n132 = Index Array(array=w380, index=w377) -> (element=w379:string)
        n133 = To Variant(anything=w379) -> (Variant=w383:variant)
        n134 = Bundle By Name(cluster=T4 {"State"="", "Data"=variant} ("State_and_Data"), "State"="Update_Wash", "Data"=w383) -> (w385:T4)
        n135 = call "QD_Washing_Machine.vi"("Data_In"=w385, "Error_In"=w381, "Queue_Operation_Select"=w387) -> ("Error_Out"=w374:errorcluster)  [unwired: 10 in, 2 out]
      }
      event "Start_Wash": Value Change {
        w394 = Queue_Operation_Select."Enqueue"  # Queue_Operation_Select
        # "Add the clothes to machine"
        n136 = event-data() -> ()  [unwired: 1 in, 1 out]
        n137 = Bundle By Name(cluster=T4 {"State"="", "Data"=variant} ("State_and_Data"), "State"="Start") -> (w392:T4)
        n138 = call "QD_Washing_Machine.vi"("Data_In"=w392, "Error_In"=w396, "Queue_Operation_Select"=w394) -> ("Error_Out"=w395:errorcluster)  [unwired: 10 in, 2 out]
      }
      event "Stop_Wash": Value Change {
        w403 = Queue_Operation_Select."Enqueue"  # Queue_Operation_Select
        # "Request to stop the washing process"
        n139 = event-data() -> ()  [unwired: 1 in, 1 out]
        n140 = Bundle By Name(cluster=T4 {"State"="", "Data"=variant} ("State_and_Data"), "State"="Stop_Washing") -> (w401:T4)
        n141 = call "QD_Washing_Machine.vi"("Data_In"=w401, "Error_In"=w404, "Queue_Operation_Select"=w403) -> ("Error_Out"=w398:errorcluster)  [unwired: 10 in, 2 out]
      }
      event "Unload": Value Change {
        w410 = Queue_Operation_Select."Enqueue"  # Queue_Operation_Select
        # "Request for Unload of clothes"
        n142 = event-data() -> ()  [unwired: 1 in, 1 out]
        n143 = Bundle By Name(cluster=T4 {"State"="", "Data"=variant} ("State_and_Data"), "State"="Unload") -> (w408:T4)
        n144 = call "QD_Washing_Machine.vi"("Data_In"=w408, "Error_In"=w412, "Queue_Operation_Select"=w410) -> ("Error_Out"=w411:errorcluster)  [unwired: 10 in, 2 out]
      }
      event Panel Close? {
        w419 = Queue_Operation_Select."Enqueue"  # Queue_Operation_Select
        # "Handles the panel close"
        n145 = event-data() -> ()  [unwired: 1 in, 2 out]
        n146 = Bundle By Name(cluster=T4 {"State"="", "Data"=variant} ("State_and_Data"), "State"="Exit") -> (w417:T4)
        n147 = call "QD_Washing_Machine.vi"("Data_In"=w417, "Error_In"=w421, "Queue_Operation_Select"=w419) -> ("Error_Out"=w420:errorcluster)  [unwired: 10 in, 2 out]
        n148 = event-data ("Event Filter Node")("Discard?"=TRUE) -> ()  [unwired: 1 in, 1 out]
      }
      event User Event {
        # "Close the application"
        n149 = event-data() -> ("Exit"=w422:bool)  [unwired: 1 in]
      }
    }
  }
  n150 = Merge Errors(w23, w16) -> (w9:errorcluster)
  n151 = Unregister For Events(event registration refnum=w1, error in=w9) -> (error out=w2:errorcluster)
  n152 = Destroy User Event(user event=w3, error in=w2) -> (error out=w10:errorcluster)
  n153 = call "QD_Washing_Machine.vi"("Error_In"=w10, "Queue_Operation_Select"=w6) -> ("Error_Out"=w7:errorcluster)  [unwired: 11 in, 2 out]
  n154 = call "QD_Washing_Machine.vi"("Error_In"=w7, "Queue_Operation_Select"=w5) -> ("Error_Out"=→"Error_Out":errorcluster)  [unwired: 11 in, 2 out]
